vi "AndorPhysikInstrumenteInitialisiation.vi"(7 "reference":refnum<vi>, 8 "error in (no error)":errorcluster, 9 "reference 3":refnum<vi>, 10 "reference 2":refnum<vi>, 11 "Pi":i32) -> (0 "error out":errorcluster, 3 "Device List":T1(array[cluster]))   [LabVIEW 2011]
uses:
  Variables/GlobalConAxisPI.vi
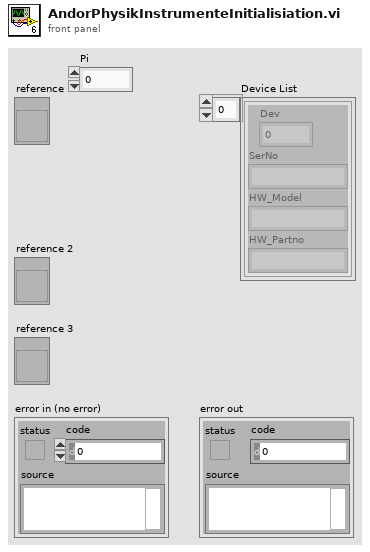
[diagram p1: front panel]
types:
  T1 = cluster{"Dev":i32, "SerNo":string, "HW_Model":string, "HW_Partno":string}[]
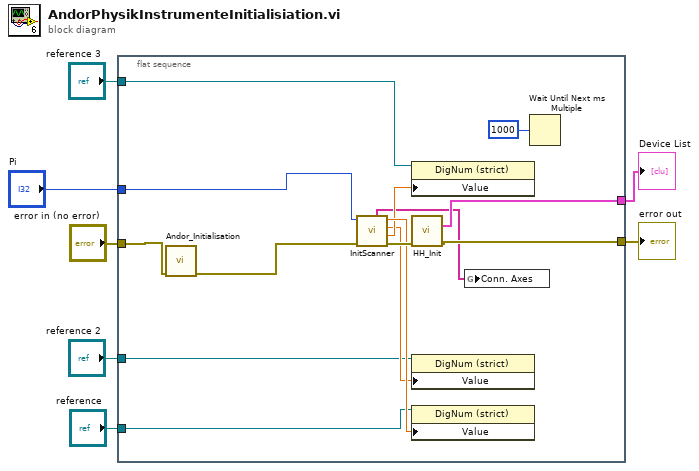
[diagram p0: block diagram]
diagram:
  n1 = flat-sequence {
    tunnel: [w21] -> w5
    tunnel: "error in (no error)" -> [w16]
    tunnel: [w10] -> w7
    tunnel: "reference" -> [w13]
    tunnel: "reference 2" -> [w12]
    tunnel: "reference 3" -> [w11]
    tunnel: "Pi" -> [w9]
    frame #0 {
      n2 = call "Andor_Initialisation.vi"("error in (no error)"=w16) -> ("error out"=w15:errorcluster)  [unwired: 10 in]
      n3 = call "InitScanner.vi"("error in (no error)"=w15, "PI SystemNumber"=w9) -> ("error out"=w20:errorcluster, "z-position"=w18:dbl, "y-position"=w17:dbl, "x-position"=w19:dbl, "Conn. Axes"=w8:string[])  [unwired: 5 in]
      n4 = property class="DigNum (strict)"(reference=w11, "Value"=w18) -> ()  [unwired: 1 in, 2 out]
      n5 = call "HH_Init.vi"("error in (no error)"=w20) -> ("Device List"=w21:T1, "error out"=w10:errorcluster)  [unwired: 12 in, 1 out]
      n6 = property class="DigNum (strict)"(reference=w12, "Value"=w17) -> ()  [unwired: 1 in, 2 out]
      n7 = property class="DigNum (strict)"(reference=w13, "Value"=w19) -> ()  [unwired: 1 in, 2 out]
      n8 = global write "GlobalConAxisPI.vi" "Conn. Axes"(w8) -> ()
      n9 = Wait Until Next ms Multiple(millisecond multiple=u32 1000) -> ()  [unwired: 1 out]
    }
  }
  "error out" <- w7
  "Device List" <- w5
